vi "Get Trigger Count.vi"(8 "error in":errorcluster, 11 "VISA resource name in":refnum<visa-resource-name>) -> (0 "error out":errorcluster, 2 "Count":dbl, 3 "VISA resource name out":refnum<visa-resource-name>)   [LabVIEW 2021, in "Keysight U1282A.lvlib"]
doc: "El comando de obtener el conteo de disparo (TRIG:REF:COUN?) regresa el conteo del modo auto hold."
uses:
  Keysight U1282A.lvlib
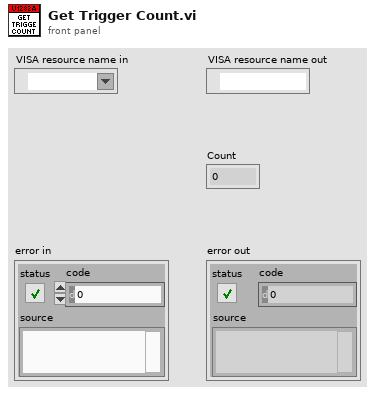
[diagram p1: front panel]
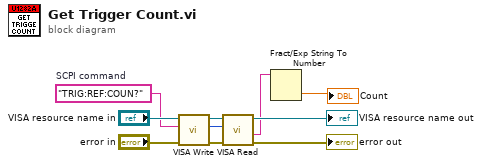
[diagram p0: block diagram]
diagram:
  w3 = "TRIG:REF:COUN?"  # SCPI command
  n1 = call "VISA Write.vi"("error in"="error in", "SCPI command"=w3, "VISA resource in"="VISA resource name in") -> ("error out"=w10:errorcluster, "Bytes at Port out"=w8:u32, "VISA resource out"=w9:refnum<visa-resource-name>)  [unwired: 6 in]
  n2 = call "VISA Read.vi"("error in"=w10, "Bytes at Port in"=w8, "VISA resource in"=w9) -> ("error out"=→"error out":errorcluster, "Reading"=w2:string, "VISA resource out"=→"VISA resource name out":refnum<visa-resource-name>)  [unwired: 5 in, 1 out]
  n3 = Fract/Exp String To Number(string=w2) -> (number=→"Count":dbl)  [unwired: 3 in, 1 out]
